vi "Init_Simple_Var.vi"(4 "Value":T1) -> (1 "Var":refnum<class "Var_Str.lvclass">)   [LabVIEW 2021, in "Var_Str.lvclass"]
uses:
  Var_Str.lvclass
  Type.ctl
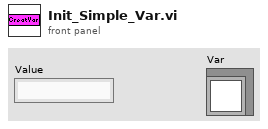
[diagram p1: front panel]
types:
  T1 = typedef "Var_Str.lvclass/Type.ctl" = string
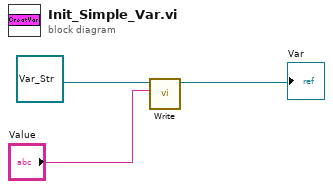
[diagram p0: block diagram]
diagram:
  n1 = call-dynamic "Write.vi"("Value"="Value", "Double Float.lvclass_340760 in"=refnum<class "Var_Str.lvclass"> refnum ("Constants.lvlib:Numeric.lvclass")) -> ("Double Float.lvclass_340760 out"=→"Var":refnum<class "Var_Str.lvclass">)  [unwired: 8 in, 1 out]
